vi "Get BuildWorker Default Configuration.vi"(8 "error in (no error)":errorcluster, 10 "configuration file path":path, 11 "BuildWorker in":refnum<class "BuildWorker.lvclass">) -> (0 "error out":errorcluster, 2 "#Max Worker":i32, 3 "BuildWorker out":refnum<class "BuildWorker.lvclass">)   [LabVIEW 2017, in "BuildWorker Interface.lvlib" / "BuildWorker.lvclass"]
uses:
  BuildWorker.lvclass
  BuildWorker.lvclass/BuildWorker.ctl
  <vilib>/Utility/config.llb/Read Key (String).vi
  <vilib>/Utility/config.llb/Read Key (Path).vi
  <vilib>/Utility/config.llb/Read Key (Boolean).vi
  <vilib>/Utility/config.llb/Read Key (U32).vi
  <vilib>/Utility/config.llb/NI_LVConfig.lvlib
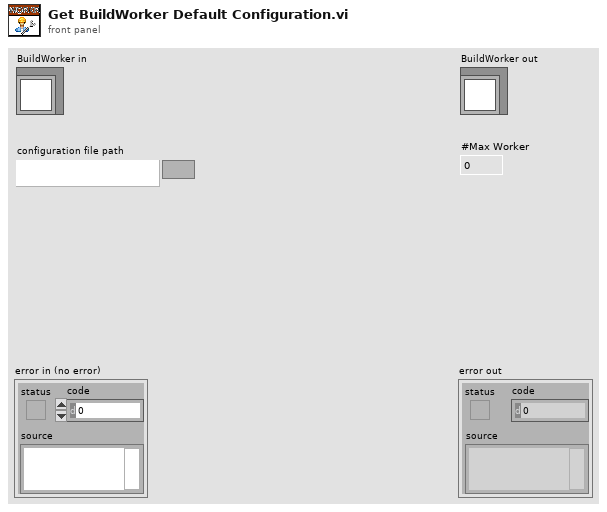
[diagram p1: front panel]
types:
  T1 = typedef "NI_LVConfig.lvlib/Config Data RefNum.ctl" = refnum<k1>
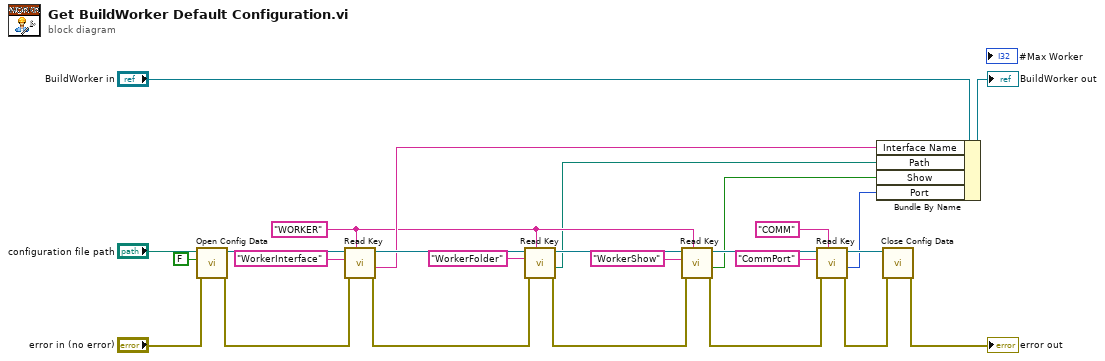
[diagram p0: block diagram]
diagram:
  w4 = "WORKER" ("section")
  n1 = call <vilib>:"Open Config Data.vi"("error in (no error)"="error in (no error)", "create file if necessary (T)"=FALSE, "configuration file path"="configuration file path") -> ("error out"=w24:errorcluster, "refnum"=w25:T1)  [unwired: 6 in, 1 out]
  n2 = call-poly <vilib>:"Read Key.vi"("section"=w4, "error in (no error)"=w24, "key"="WorkerInterface", "refnum"=w25) -> ("error out"=w7:errorcluster, "value"=w5:string, "refnum out"=w10:T1)  [unwired: 4 in, 1 out]
  n3 = call-poly <vilib>:"Read Key.vi"("section"=w4, "error in (no error)"=w7, "key"="WorkerFolder", "refnum"=w10) -> ("error out"=w6:errorcluster, "value"=w3:path, "refnum out"=w9:T1)  [unwired: 4 in, 1 out]
  n4 = call-poly <vilib>:"Read Key.vi"("section"=w4, "error in (no error)"=w6, "key"="WorkerShow", "refnum"=w9) -> ("error out"=w18:errorcluster, "value"=w11:bool, "refnum out"=w19:T1)  [unwired: 4 in, 1 out]
  n5 = call-poly <vilib>:"Read Key.vi"("section"="COMM", "error in (no error)"=w18, "key"="CommPort", "refnum"=w19) -> ("error out"=w16:errorcluster, "value"=w14:u32, "refnum out"=w17:T1)  [unwired: 4 in, 1 out]
  n6 = Bundle By Name(cluster="BuildWorker in", "Interface Name"=w5, "Path"=w3, "Show"=w11, "Port"=w14) -> (→"BuildWorker out":refnum<class "BuildWorker.lvclass">)
  n7 = call <vilib>:"Close Config Data.vi"("error in (no error)"=w16, "refnum"=w17) -> ("error out"=→"error out":errorcluster)  [unwired: 8 in, 1 out]
